vi "CheckValueEqualsSetpoint.vi"(9 "Pressure tolerance %":sgl, 10 "PressureNewVal":sgl, 11 "Device Data":T1 {"IDS" format="%.0x"; "IDL" format="%.0x"; "IDM" format="%.0x"; "IDH" format="%.0x"}) -> (0 "Current pressure status":string, 1 "Unit":string, 2 "Pressure":sgl, 3 "Function Output Comment":string, 4 "Message":string, 5 "PeqPSet ?":bool)   [LabVIEW 2019]
uses:
  Device Data.ctl
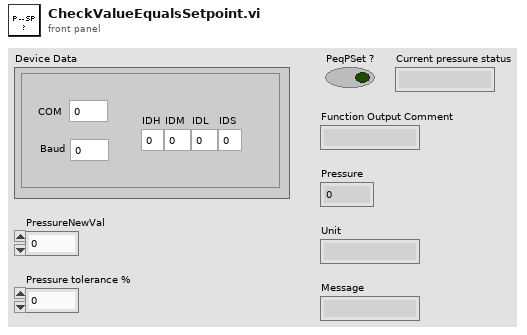
[diagram p1: front panel]
types:
  T1 = typedef "Device Data.ctl" = cluster{"COM":i32, "Baud":i32, "IDH":u8, "IDM":u8, "IDL":u8, "IDS":u8}
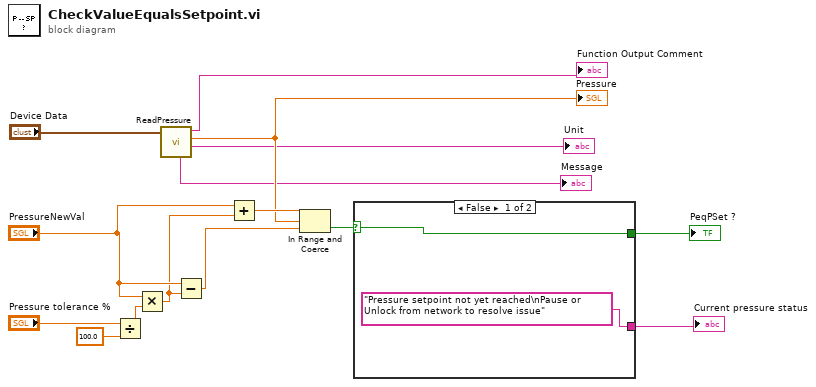
[diagram p0: block diagram]
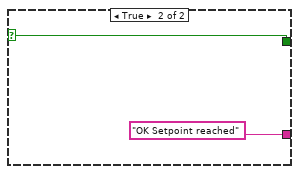
[diagram p2: hidden frame]
diagram:
  n1 = Divide(x="Pressure tolerance %", y=sgl 100.0) -> (x/y=w9:sgl)
  n2 = Multiply(x="PressureNewVal", y=w9) -> (x*y=w12:sgl)
  n3 = call "ReadPressure.vi"("Device Data"="Device Data") -> ("Unit"=→"Unit":string, "Pressure"=w8:sgl, "Function Output Comment"=→"Function Output Comment":string, "Message"=→"Message":string)  [unwired: 7 in]
  "Pressure" <- w8
  n4 = Subtract(x="PressureNewVal", y=w12) -> (x-y=w15:sgl)
  n5 = Add(x="PressureNewVal", y=w12) -> (x+y=w14:sgl)
  n6 = In Range and Coerce(upper limit=w14, x=w8, lower limit=w15) -> (In Range?=w3:bool)  [unwired: 1 out]
  n7 = case shown="False" w3 {
    selector: w3 -> [w17 w19]
    tunnel: [w17 w19] -> w2
    tunnel: ["Pressure setpoint not yet reached\nPause or Unlock from network to resolve issue" ("Current pressure status") "OK Setpoint reached" ("Current pressure status")] -> w1
    frame False {
    }
    frame True {
    }
  }
  "PeqPSet ?" <- w2
  "Current pressure status" <- w1
